vi "Quiz11.vi"() -> ()   [LabVIEW 2017]
panel:
  out "มากไปน้อย":i8[](array[numeric])
  out "เรียงจากน้อยไปมาก":i8[](array[numeric])
  out "min index(es)":i32
  out "min value":i8
  out "max index(es)":i32
  out "max value":i8
  out "สุ่ม":i8[](array[numeric])
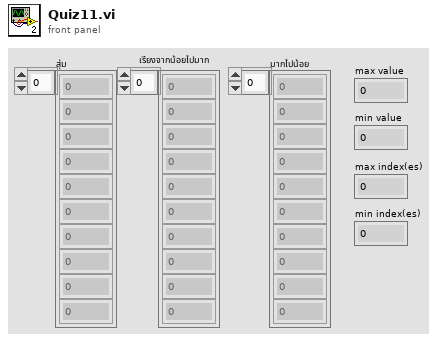
[diagram p1: front panel]
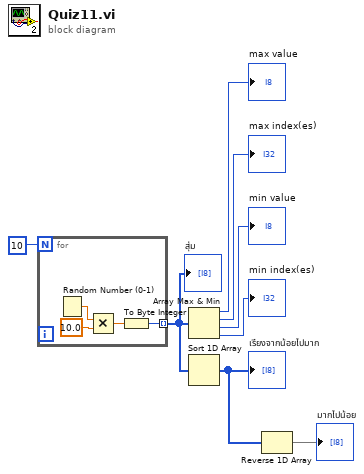
[diagram p0: block diagram]
diagram:
  n1 = for {
    N: 10 -> [_]
    tunnel: [w9] -> w3 mode=indexing
    n2 = Random Number (0-1)() -> (number: 0 to 1=w12:dbl)
    n3 = Multiply(x=w12, y=10.0) -> (x*y=w10:dbl)
    n4 = To Byte Integer(number=w10) -> (8bit integer=w9:i8)
  }
  "สุ่ม" <- w3
  n5 = Array Max & Min(array=w3) -> (max value=→"max value":i8, max index (indices)=→"max index(es)":i32, min value=→"min value":i8, min index (indices)=→"min index(es)":i32)
  n6 = Sort 1D Array(array=w3) -> (sorted array=w2:i8[])
  "เรียงจากน้อยไปมาก" <- w2
  n7 = Reverse 1D Array(array=w2) -> (reversed array=→"มากไปน้อย":i8[])
